vi "user32_UpdateWindow.vi"(8 "错误输入（无错误）":errorcluster, 11 "hWnd":u32) -> (0 "错误输出":errorcluster, 2 "success?":bool, 3 "dup hWnd":u32)   [LabVIEW 2011]
doc: "如果窗口更新的区域不为空，UpdateWindow函数通过发送一个WM_PAINT消息来更新指定窗口的客户区。函数绕过应用程序的消息队列，直接发送WM_PAINT消息给指定窗口的窗口过程，如果更新区域为空，则不发送消息。"
uses:
  user32.dll
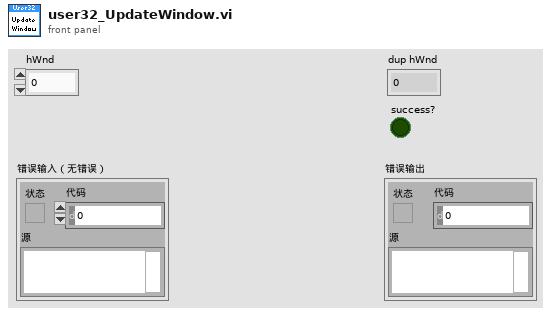
[diagram p1: front panel]
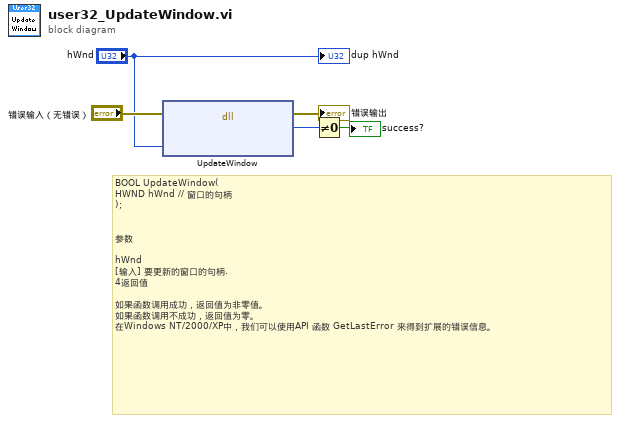
[diagram p0: block diagram]
diagram:
  # "BOOL UpdateWindow(\nHWND hWnd // 窗口的句柄\n);\n\n\n参数\n\nhWnd\n[输入] 要更新的窗口的句柄.\n4返回值\n\n如果函数调用成功，返回值为非零值。\n如果函数调用不成功，返回值为零。\n在Windows NT/2000/XP中，我们可以使用API 函数 GetLastError 来得到扩展的错误信息。"
  n1 = dll-call lib="user32.dll" fn="UpdateWindow"(error in="错误输入（无错误）", "hWnd"="hWnd") -> (error out=→"错误输出":errorcluster, "Bool"=w2:i32)  [unwired: 3 in, 1 out]
  n2 = Not Equal To 0?(x=w2) -> (x != 0?=→"success?":bool)
  "dup hWnd" <- "hWnd"
